vi "Update Data.vi"(8 "error in":errorcluster, 10 "Data":T1, 11 "CutomOOB_Tx in":refnum<class "TemplateOOB_Tx.lvclass">) -> (0 "error out":errorcluster, 3 "CutomOOB_Tx out":refnum<class "TemplateOOB_Tx.lvclass">)   [LabVIEW 2021, in "TemplateOOB_Tx.lvclass"]
uses:
  TemplateOOB_Tx.lvclass
  TemplateOOB_Tx.lvclass/TemplateOOB_Tx.ctl
  <vilib>/CIF Foundation/CIF Out of Band Commands/CIFOutOfBand.lvclass
  Typedef/OOB Commands.ctl
  Typedef/Payload.ctl
  Typedef/Main to gRPC Command Data.ctl
  <vilib>/CIF Foundation/CIF Out of Band Commands/Typedef/OOB Container.ctl
  C:/Program Files/National Instruments/LabVIEW 2021/vi.lib/CIF Foundation/CIF Out of Band Commands/CIFOutOfBand.lvclass
  D:/dev/Plugins/Template/OOB/OOB_Tx/TemplateOOB_Tx.lvclass
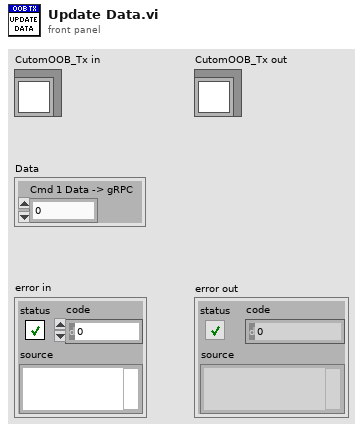
[diagram p1: front panel]
types:
  T1 = typedef "TemplateOOB_Tx.lvclass/Main to gRPC Command Data.ctl" = cluster{"Cmd 1 Data -> gRPC":i32}
  T2 = typedef "CIFOutOfBand.lvclass/OOB Container.ctl" = cluster{"Commands (bitwise)":u64, "Payload":variant}
  T3 = typedef "TemplateOOB_Tx.lvclass/Payload.ctl" = cluster{"Data":T1}
  T4 = typedef "TemplateOOB_Tx.lvclass/OOB Commands.ctl" = enum8{"Command 1"}
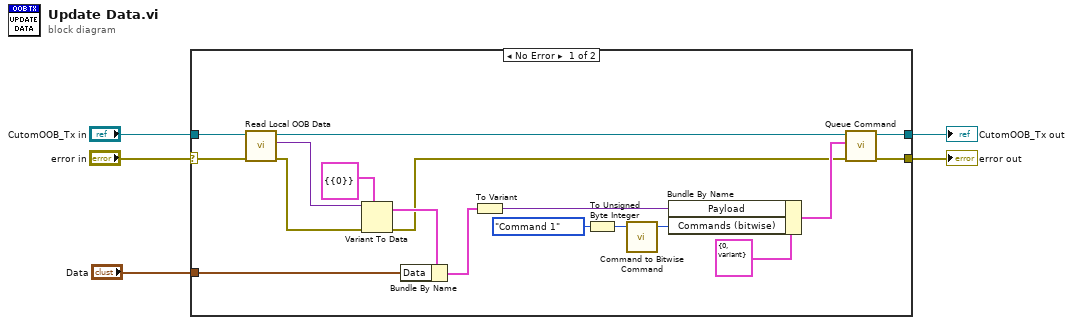
[diagram p0: block diagram]
diagram:
  n1 = case shown="No Error" "error in" {
    selector: "error in" -> [w13 w25]
    tunnel: [w22 w25] -> w4
    tunnel: "CutomOOB_Tx in" -> [w14 w24]
    tunnel: [w23 w24] -> w2
    tunnel: "Data" -> [w12 _]
    frame No Error {
      n2 = call <vilib>:"Read Local OOB Data.vi"("error in"=w13, "OOB in"=w14) -> ("error out"=w16:errorcluster, "Local OOB Data"=w19:variant, "OOB out"=w7:refnum<class "TemplateOOB_Tx.lvclass">)  [unwired: 7 in]
      n3 = Variant To Data(error in=w16, type=T3 {"Data"={"Cmd 1 Data -> gRPC"=0}} ("Template Payload"), Variant=w19) -> (data=w17:T3, error out=w8:errorcluster)
      n4 = Bundle By Name(cluster=w17, "Data"=w12) -> (w15:T3)
      n5 = To Variant(anything=w15) -> (Variant=w6:variant)
      n6 = To Unsigned Byte Integer(number=OOB_Commands."Command 1" ("OOB Main Commands")) -> (unsigned 8bit integer=w21:u8)
      n7 = call <vilib>:"Command to Bitwise Command.vi"("Command"=w21) -> ("bit command"=w10:u64)  [unwired: 3 in]
      n8 = Bundle By Name(cluster=T2 {"Commands (bitwise)"=0, "Payload"=variant} ("OOB Data"), "Payload"=w6, "Commands (bitwise)"=w10) -> (w9:T2)
      n9 = call <vilib>:"Queue Command.vi"("error in"=w8, "OOB Data"=w9, "OOB in"=w7) -> ("error out"=w22:errorcluster, "OOB out"=w23:refnum<class "TemplateOOB_Tx.lvclass">)  [unwired: 7 in]
    }
    frame Error {
    }
  }
  "error out" <- w4
  "CutomOOB_Tx out" <- w2
